vi "test-Coordinate-System-Test1.vi"() -> (3 "All tests passed":bool)   [LabVIEW 2019]
uses:
  <vilib>/Rock Robotics/WPI/ThirdParty/JAS_Junk/TrajLib/CoordAxis_N.vi
  <vilib>/Rock Robotics/WPI/ThirdParty/JAS_Junk/TrajLib/CoordAxis_W.vi
  <vilib>/Rock Robotics/WPI/ThirdParty/JAS_Junk/TrajLib/CoordAxis_U.vi
  <vilib>/Rock Robotics/WPI/ThirdParty/JAS_Junk/TrajLib/CoordSystem_New.vi
  <vilib>/Rock Robotics/WPI/ThirdParty/JAS_Junk/TrajLib/CoordAxis_E.vi
  <vilib>/Rock Robotics/WPI/ThirdParty/JAS_Junk/TrajLib/CoordAxis_D.vi
  <vilib>/Rock Robotics/WPI/ThirdParty/JAS_Junk/TrajLib/Conv_Deg_Radians.vi
  <vilib>/Rock Robotics/WPI/ThirdParty/JAS_Junk/TrajLib/Quaternion_New.vi
  <vilib>/Rock Robotics/WPI/ThirdParty/JAS_Junk/TrajLib/Translation3d_Create.vi
  <vilib>/Rock Robotics/WPI/ThirdParty/JAS_Junk/TrajLib/Pose3d_New_Trans3dRot3d.vi
  <vilib>/Rock Robotics/WPI/ThirdParty/JAS_Junk/TrajLib/Rotation3d_Minus.vi
  <vilib>/Rock Robotics/WPI/ThirdParty/JAS_Junk/TrajLib/Translation3d_Create_Default.vi
  <vilib>/Rock Robotics/WPI/ThirdParty/JAS_Junk/TrajLib/Pose3d_RelativeTo.vi
  <vilib>/Rock Robotics/WPI/ThirdParty/JAS_Junk/TrajLib/Translation3d_Equals.vi
  <vilib>/Rock Robotics/WPI/ThirdParty/JAS_Junk/TrajLib/Rotation3d_Equals.vi
  <vilib>/Rock Robotics/WPI/ThirdParty/JAS_Junk/TrajLib/Pose3d_getTranslation3d.vi
  <vilib>/Rock Robotics/WPI/ThirdParty/JAS_Junk/TrajLib/Pose3d_getRotation3d.vi
  <vilib>/Rock Robotics/WPI/ThirdParty/JAS_Junk/TrajLib/CoordAxis_New.vi
  <vilib>/Rock Robotics/WPI/ThirdParty/JAS_Junk/TrajLib/MatBuilder_Create.vi
  <vilib>/Rock Robotics/WPI/ThirdParty/JAS_Junk/TrajLib/Matrix_AssignBlock.vi
  <vilib>/Rock Robotics/WPI/ThirdParty/JAS_Junk/TrajLib/Matrix_Transpose.vi
  <vilib>/Rock Robotics/WPI/ThirdParty/JAS_Junk/TrajLib/Matrix_Ident.vi
  <vilib>/Rock Robotics/WPI/ThirdParty/JAS_Junk/TrajLib/Matrix_IsEqual.vi
  <vilib>/Analysis/baseanly.llb/A x B.vi
  <vilib>/Analysis/baseanly.llb/Real A x B.vi
  <vilib>/Rock Robotics/WPI/ThirdParty/JAS_Junk/TrajLib/Rotation3d_Create_Quaternion.vi
  <vilib>/Rock Robotics/WPI/ThirdParty/JAS_Junk/TrajLib/Rotation3d_UnaryMinus.vi
  <vilib>/Rock Robotics/WPI/ThirdParty/JAS_Junk/TrajLib/Rotation3d_RotateBy.vi
  <vilib>/Rock Robotics/WPI/ThirdParty/JAS_Junk/TrajLib/Transform3d_Create_Pose3dPose3d.vi
  <vilib>/Rock Robotics/WPI/ThirdParty/JAS_Junk/TrajLib/Transform3d_GetRotation3d.vi
  <vilib>/Rock Robotics/WPI/ThirdParty/JAS_Junk/TrajLib/Transform3d_GetTranslation3d.vi
  <vilib>/Rock Robotics/WPI/ThirdParty/JAS_Junk/TrajLib/Rotation3d_GetQuaterion.vi
  <vilib>/Rock Robotics/WPI/ThirdParty/JAS_Junk/TrajLib/Quaternion_Equals.vi
  <vilib>/Rock Robotics/WPI/ThirdParty/JAS_Junk/TrajLib/MatrixHelper_CoerceSize.vi
  <vilib>/Rock Robotics/WPI/ThirdParty/JAS_Junk/TrajLib/Quaternion_Normalize.vi
  <vilib>/Rock Robotics/WPI/ThirdParty/JAS_Junk/TrajLib/Quaternion_Inverse.vi
  <vilib>/Rock Robotics/WPI/ThirdParty/JAS_Junk/TrajLib/Quaternion_Times.vi
  <vilib>/Rock Robotics/WPI/ThirdParty/JAS_Junk/TrajLib/Transform3d_Create_Trans3dRot3d.vi
  <vilib>/Rock Robotics/WPI/ThirdParty/JAS_Junk/TrajLib/Translation3d_Minus.vi
  <vilib>/Rock Robotics/WPI/ThirdParty/JAS_Junk/TrajLib/Translation3d_RotateBy.vi
  <vilib>/Rock Robotics/WPI/ThirdParty/JAS_Junk/TrajLib/Quaternion_New_Default.vi
  <vilib>/Rock Robotics/WPI/ThirdParty/JAS_Junk/TrajLib/Quaternion_Get_All.vi
  <vilib>/Analysis/7linalg.llb/Create Special Matrix.vi
  <vilib>/Analysis/7linalg.llb/Create Special Real Matrix.vi
  <vilib>/Analysis/Matrix/Numeric/Conversions/Array To Matrix.vi
  <vilib>/Analysis/Matrix/Numeric/Conversions/Array To Matrix - RA.vi
  <vilib>/Rock Robotics/WPI/ThirdParty/JAS_Junk/TrajLib/Trajectory_Library.lvlib
panel:
  out "Test 4":bool
  out "Test 3":bool
  out "Test 2":bool
  out "Test 1":bool
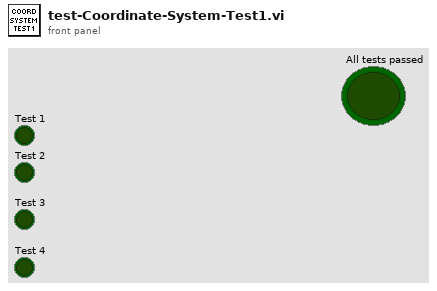
[diagram p1: front panel]
types:
  T1 = typedef "Trajectory_Library.lvlib/ROTATION3D.ctl" = cluster{"Q_quaternion":T2}
  T2 = typedef "Trajectory_Library.lvlib/QUATERNION.ctl" = cluster{"R":dbl, "V":dbl[]}
  T3 = typedef "Trajectory_Library.lvlib/POSE3D.ctl" = cluster{"Translation3d":T4, "Rotation3d":T1}
  T4 = typedef "Trajectory_Library.lvlib/TRANSLATION3D.ctl" = cluster{"X":dbl, "Y":dbl, "Z":dbl}
  T5 = typedef "Trajectory_Library.lvlib/COORDINATE_SYSTEM.ctl" = cluster{"Rotation":T1}
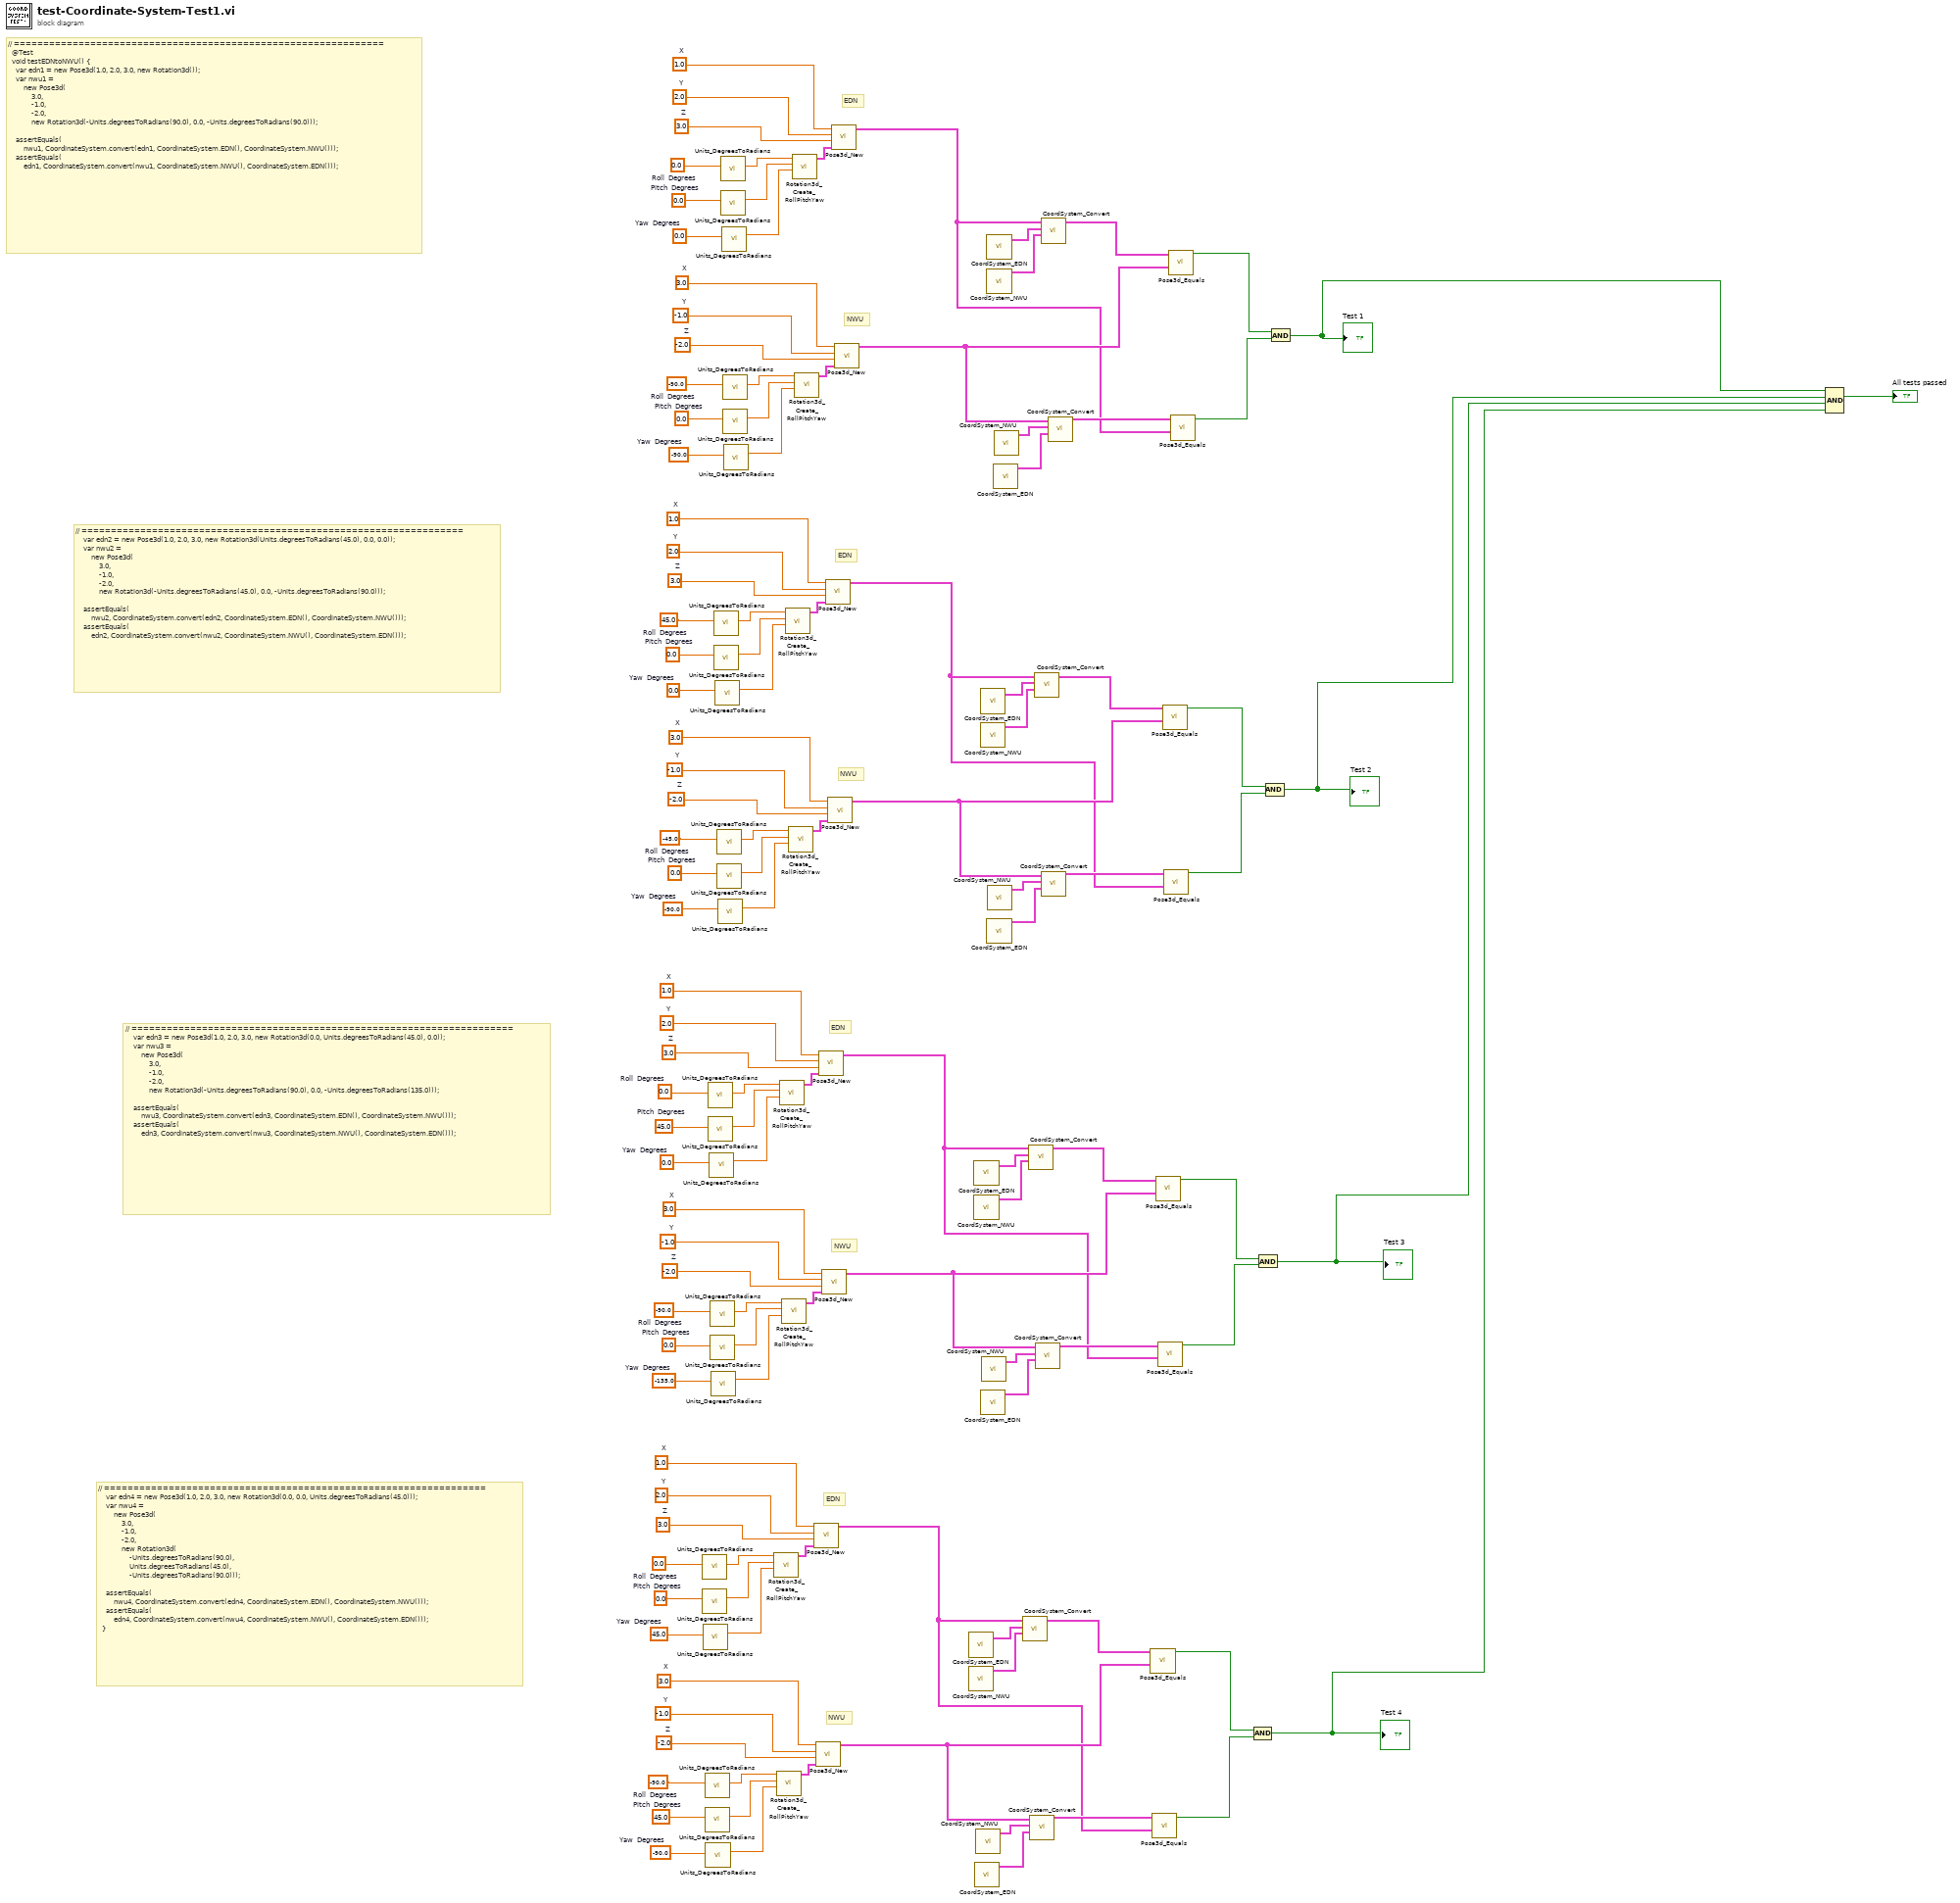
[diagram p0: block diagram]
diagram:
  w22 = 3.0  # X
  w21 = -1.0  # Y
  w20 = -2.0  # Z
  w14 = -90.0  # Roll  Degrees
  w15 = 45.0  # Pitch  Degrees
  w16 = -90.0  # Yaw  Degrees
  w32 = 1.0  # X
  w31 = 2.0  # Y
  w30 = 3.0  # Z
  w24 = 0.0  # Roll  Degrees
  w25 = 0.0  # Pitch  Degrees
  w26 = 45.0  # Yaw  Degrees
  w52 = 3.0  # X
  w51 = -1.0  # Y
  w50 = -2.0  # Z
  w44 = -90.0  # Roll  Degrees
  w45 = 0.0  # Pitch  Degrees
  w46 = -135.0  # Yaw  Degrees
  w62 = 1.0  # X
  w61 = 2.0  # Y
  w60 = 3.0  # Z
  w54 = 0.0  # Roll  Degrees
  w55 = 45.0  # Pitch  Degrees
  w56 = 0.0  # Yaw  Degrees
  w82 = 3.0  # X
  w81 = -1.0  # Y
  w80 = -2.0  # Z
  w74 = -45.0  # Roll  Degrees
  w75 = 0.0  # Pitch  Degrees
  w76 = -90.0  # Yaw  Degrees
  w92 = 1.0  # X
  w91 = 2.0  # Y
  w90 = 3.0  # Z
  w84 = 45.0  # Roll  Degrees
  w85 = 0.0  # Pitch  Degrees
  w86 = 0.0  # Yaw  Degrees
  w114 = 3.0  # X
  w113 = -1.0  # Y
  w112 = -2.0  # Z
  w106 = -90.0  # Roll  Degrees
  w107 = 0.0  # Pitch  Degrees
  w108 = -90.0  # Yaw  Degrees
  w124 = 1.0  # X
  w123 = 2.0  # Y
  w122 = 3.0  # Z
  w116 = 0.0  # Roll  Degrees
  w117 = 0.0  # Pitch  Degrees
  w118 = 0.0  # Yaw  Degrees
  # "// =================================================================\n    var edn2 = new Pose3d(1.0, 2.0, 3.0, new Rotation3d(Units.degreesToRadians(45.0), 0.0, 0.0));\n    var nwu2 =\n        new Pose3d(\n            3.0,\n            -1.0,\n            -2.0,\n            new Rotation3d(-Units.degreesToRadians(45.0), 0.0, -Units.degreesToRadians(90.0)));\n\n    assertEquals(\n        nwu2, CoordinateSystem.convert(edn2, CoordinateSystem.EDN(), CoordinateSystem.NWU()));\n    assertEquals(\n        edn2, CoordinateSystem.convert(nwu2, CoordinateSystem.NWU(), CoordinateSystem.EDN()));"
  # "// =================================================================\n    var edn3 = new Pose3d(1.0, 2.0, 3.0, new Rotation3d(0.0, Units.degreesToRadians(45.0), 0.0));\n    var nwu3 =\n        new Pose3d(\n            3.0,\n            -1.0,\n            -2.0,\n            new Rotation3d(-Units.degreesToRadians(90.0), 0.0, -Units.degreesToRadians(135.0)));\n\n    assertEquals(\n        nwu3, CoordinateSystem.convert(edn3, CoordinateSystem.EDN(), CoordinateSystem.NWU()));\n    assertEquals(\n        edn3, CoordinateSystem.convert(nwu3, CoordinateSystem.NWU(), CoordinateSystem.EDN()));"
  # "// =================================================================\n    var edn4 = new Pose3d(1.0, 2.0, 3.0, new Rotation3d(0.0, 0.0, Units.degreesToRadians(45.0)));\n    var nwu4 =\n        new Pose3d(\n            3.0,\n            -1.0,\n            -2.0,\n            new Rotation3d(\n                -Units.degreesToRadians(90.0),\n                Units.degreesToRadians(45.0),\n                -Units.degreesToRadians(90.0)));\n\n    assertEquals(\n        nwu4, CoordinateSystem.convert(edn4, CoordinateSystem.EDN(), CoordinateSystem.NWU()));\n    assertEquals(\n        edn4, CoordinateSystem.convert(nwu4, CoordinateSystem.NWU(), CoordinateSystem.EDN()));\n  }"
  # "NWU"
  # "EDN"
  # "NWU"
  # "EDN"
  # "NWU"
  # "EDN"
  # "NWU"
  # "EDN"
  # "// ===============================================================\n  @Test\n  void testEDNtoNWU() {\n    var edn1 = new Pose3d(1.0, 2.0, 3.0, new Rotation3d());\n    var nwu1 =\n        new Pose3d(\n            3.0,\n            -1.0,\n            -2.0,\n            new Rotation3d(-Units.degreesToRadians(90.0), 0.0, -Units.degreesToRadians(90.0)));\n\n    assertEquals(\n        nwu1, CoordinateSystem.convert(edn1, CoordinateSystem.EDN(), CoordinateSystem.NWU()));\n    assertEquals(\n        edn1, CoordinateSystem.convert(nwu1, CoordinateSystem.NWU(), CoordinateSystem.EDN()));"
  n1 = call <vilib>:"Units_DegreesToRadians.vi"("Degrees"=w24) -> ("Radians"=w27:dbl)  [unwired: 10 in]
  n2 = call <vilib>:"Units_DegreesToRadians.vi"("Degrees"=w25) -> ("Radians"=w28:dbl)  [unwired: 10 in]
  n3 = call <vilib>:"Units_DegreesToRadians.vi"("Degrees"=w26) -> ("Radians"=w29:dbl)  [unwired: 10 in]
  n4 = call <vilib>:"Units_DegreesToRadians.vi"("Degrees"=w14) -> ("Radians"=w17:dbl)  [unwired: 10 in]
  n5 = call <vilib>:"Units_DegreesToRadians.vi"("Degrees"=w15) -> ("Radians"=w18:dbl)  [unwired: 10 in]
  n6 = call <vilib>:"Units_DegreesToRadians.vi"("Degrees"=w16) -> ("Radians"=w19:dbl)  [unwired: 10 in]
  n7 = call <vilib>:"Units_DegreesToRadians.vi"("Degrees"=w54) -> ("Radians"=w57:dbl)  [unwired: 10 in]
  n8 = call <vilib>:"Units_DegreesToRadians.vi"("Degrees"=w55) -> ("Radians"=w58:dbl)  [unwired: 10 in]
  n9 = call <vilib>:"Units_DegreesToRadians.vi"("Degrees"=w56) -> ("Radians"=w59:dbl)  [unwired: 10 in]
  n10 = call <vilib>:"Units_DegreesToRadians.vi"("Degrees"=w44) -> ("Radians"=w47:dbl)  [unwired: 10 in]
  n11 = call <vilib>:"Units_DegreesToRadians.vi"("Degrees"=w45) -> ("Radians"=w48:dbl)  [unwired: 10 in]
  n12 = call <vilib>:"Units_DegreesToRadians.vi"("Degrees"=w46) -> ("Radians"=w49:dbl)  [unwired: 10 in]
  n13 = call <vilib>:"Units_DegreesToRadians.vi"("Degrees"=w84) -> ("Radians"=w87:dbl)  [unwired: 10 in]
  n14 = call <vilib>:"Units_DegreesToRadians.vi"("Degrees"=w85) -> ("Radians"=w88:dbl)  [unwired: 10 in]
  n15 = call <vilib>:"Units_DegreesToRadians.vi"("Degrees"=w86) -> ("Radians"=w89:dbl)  [unwired: 10 in]
  n16 = call <vilib>:"Units_DegreesToRadians.vi"("Degrees"=w74) -> ("Radians"=w77:dbl)  [unwired: 10 in]
  n17 = call <vilib>:"Units_DegreesToRadians.vi"("Degrees"=w75) -> ("Radians"=w78:dbl)  [unwired: 10 in]
  n18 = call <vilib>:"Units_DegreesToRadians.vi"("Degrees"=w76) -> ("Radians"=w79:dbl)  [unwired: 10 in]
  n19 = call <vilib>:"Units_DegreesToRadians.vi"("Degrees"=w116) -> ("Radians"=w119:dbl)  [unwired: 10 in]
  n20 = call <vilib>:"Units_DegreesToRadians.vi"("Degrees"=w117) -> ("Radians"=w120:dbl)  [unwired: 10 in]
  n21 = call <vilib>:"Units_DegreesToRadians.vi"("Degrees"=w118) -> ("Radians"=w121:dbl)  [unwired: 10 in]
  n22 = call <vilib>:"Units_DegreesToRadians.vi"("Degrees"=w106) -> ("Radians"=w109:dbl)  [unwired: 10 in]
  n23 = call <vilib>:"Units_DegreesToRadians.vi"("Degrees"=w107) -> ("Radians"=w110:dbl)  [unwired: 10 in]
  n24 = call <vilib>:"Units_DegreesToRadians.vi"("Degrees"=w108) -> ("Radians"=w111:dbl)  [unwired: 10 in]
  n25 = call <vilib>:"Rotation3d_Create_RollPitchYaw.vi"("Yaw"=w29, "Pitch"=w28, "Roll"=w27) -> ("Rotation3d"=w33:T1)  [unwired: 8 in]
  n26 = call <vilib>:"Rotation3d_Create_RollPitchYaw.vi"("Yaw"=w19, "Pitch"=w18, "Roll"=w17) -> ("Rotation3d"=w23:T1)  [unwired: 8 in]
  n27 = call <vilib>:"Rotation3d_Create_RollPitchYaw.vi"("Yaw"=w59, "Pitch"=w58, "Roll"=w57) -> ("Rotation3d"=w63:T1)  [unwired: 8 in]
  n28 = call <vilib>:"Rotation3d_Create_RollPitchYaw.vi"("Yaw"=w49, "Pitch"=w48, "Roll"=w47) -> ("Rotation3d"=w53:T1)  [unwired: 8 in]
  n29 = call <vilib>:"Rotation3d_Create_RollPitchYaw.vi"("Yaw"=w89, "Pitch"=w88, "Roll"=w87) -> ("Rotation3d"=w93:T1)  [unwired: 8 in]
  n30 = call <vilib>:"Rotation3d_Create_RollPitchYaw.vi"("Yaw"=w79, "Pitch"=w78, "Roll"=w77) -> ("Rotation3d"=w83:T1)  [unwired: 8 in]
  n31 = call <vilib>:"Rotation3d_Create_RollPitchYaw.vi"("Yaw"=w121, "Pitch"=w120, "Roll"=w119) -> ("Rotation3d"=w125:T1)  [unwired: 8 in]
  n32 = call <vilib>:"Rotation3d_Create_RollPitchYaw.vi"("Yaw"=w111, "Pitch"=w110, "Roll"=w109) -> ("Rotation3d"=w115:T1)  [unwired: 8 in]
  n33 = call <vilib>:"Pose3d_New.vi"("Rotation3d"=w33, "z"=w30, "Y"=w31, "X"=w32) -> ("out Pose3d"=w6:T3)  [unwired: 7 in]
  n34 = call <vilib>:"Pose3d_New.vi"("Rotation3d"=w23, "z"=w20, "Y"=w21, "X"=w22) -> ("out Pose3d"=w8:T3)  [unwired: 7 in]
  n35 = call <vilib>:"Pose3d_New.vi"("Rotation3d"=w63, "z"=w60, "Y"=w61, "X"=w62) -> ("out Pose3d"=w36:T3)  [unwired: 7 in]
  n36 = call <vilib>:"Pose3d_New.vi"("Rotation3d"=w53, "z"=w50, "Y"=w51, "X"=w52) -> ("out Pose3d"=w38:T3)  [unwired: 7 in]
  n37 = call <vilib>:"Pose3d_New.vi"("Rotation3d"=w93, "z"=w90, "Y"=w91, "X"=w92) -> ("out Pose3d"=w66:T3)  [unwired: 7 in]
  n38 = call <vilib>:"Pose3d_New.vi"("Rotation3d"=w83, "z"=w80, "Y"=w81, "X"=w82) -> ("out Pose3d"=w68:T3)  [unwired: 7 in]
  n39 = call <vilib>:"Pose3d_New.vi"("Rotation3d"=w125, "z"=w122, "Y"=w123, "X"=w124) -> ("out Pose3d"=w98:T3)  [unwired: 7 in]
  n40 = call <vilib>:"Pose3d_New.vi"("Rotation3d"=w115, "z"=w112, "Y"=w113, "X"=w114) -> ("out Pose3d"=w100:T3)  [unwired: 7 in]
  n41 = call <vilib>:"CoordSystem_EDN.vi"() -> ("out Coordinate System"=w13:T5)  [unwired: 10 in, 1 out]
  n42 = call <vilib>:"CoordSystem_NWU.vi"() -> ("out Coordinate System"=w12:T5)  [unwired: 10 in, 1 out]
  n43 = call <vilib>:"CoordSystem_EDN.vi"() -> ("out Coordinate System"=w43:T5)  [unwired: 10 in, 1 out]
  n44 = call <vilib>:"CoordSystem_NWU.vi"() -> ("out Coordinate System"=w42:T5)  [unwired: 10 in, 1 out]
  n45 = call <vilib>:"CoordSystem_EDN.vi"() -> ("out Coordinate System"=w10:T5)  [unwired: 10 in, 1 out]
  n46 = call <vilib>:"CoordSystem_NWU.vi"() -> ("out Coordinate System"=w11:T5)  [unwired: 10 in, 1 out]
  n47 = call <vilib>:"CoordSystem_EDN.vi"() -> ("out Coordinate System"=w73:T5)  [unwired: 10 in, 1 out]
  n48 = call <vilib>:"CoordSystem_NWU.vi"() -> ("out Coordinate System"=w72:T5)  [unwired: 10 in, 1 out]
  n49 = call <vilib>:"CoordSystem_EDN.vi"() -> ("out Coordinate System"=w40:T5)  [unwired: 10 in, 1 out]
  n50 = call <vilib>:"CoordSystem_NWU.vi"() -> ("out Coordinate System"=w41:T5)  [unwired: 10 in, 1 out]
  n51 = call <vilib>:"CoordSystem_EDN.vi"() -> ("out Coordinate System"=w105:T5)  [unwired: 10 in, 1 out]
  n52 = call <vilib>:"CoordSystem_NWU.vi"() -> ("out Coordinate System"=w104:T5)  [unwired: 10 in, 1 out]
  n53 = call <vilib>:"CoordSystem_EDN.vi"() -> ("out Coordinate System"=w70:T5)  [unwired: 10 in, 1 out]
  n54 = call <vilib>:"CoordSystem_NWU.vi"() -> ("out Coordinate System"=w71:T5)  [unwired: 10 in, 1 out]
  n55 = call <vilib>:"CoordSystem_EDN.vi"() -> ("out Coordinate System"=w102:T5)  [unwired: 10 in, 1 out]
  n56 = call <vilib>:"CoordSystem_NWU.vi"() -> ("out Coordinate System"=w103:T5)  [unwired: 10 in, 1 out]
  n57 = call <vilib>:"CoordSystem_Convert.vi"("CoordSys To"=w12, "CoordSys From"=w13, "in Pose3d"=w6) -> ("out Converted Pose3d"=w9:T3)  [unwired: 8 in]
  n58 = call <vilib>:"CoordSystem_Convert.vi"("CoordSys To"=w42, "CoordSys From"=w43, "in Pose3d"=w36) -> ("out Converted Pose3d"=w39:T3)  [unwired: 8 in]
  n59 = call <vilib>:"CoordSystem_Convert.vi"("CoordSys To"=w10, "CoordSys From"=w11, "in Pose3d"=w8) -> ("out Converted Pose3d"=w7:T3)  [unwired: 8 in]
  n60 = call <vilib>:"CoordSystem_Convert.vi"("CoordSys To"=w72, "CoordSys From"=w73, "in Pose3d"=w66) -> ("out Converted Pose3d"=w69:T3)  [unwired: 8 in]
  n61 = call <vilib>:"CoordSystem_Convert.vi"("CoordSys To"=w40, "CoordSys From"=w41, "in Pose3d"=w38) -> ("out Converted Pose3d"=w37:T3)  [unwired: 8 in]
  n62 = call <vilib>:"CoordSystem_Convert.vi"("CoordSys To"=w104, "CoordSys From"=w105, "in Pose3d"=w98) -> ("out Converted Pose3d"=w101:T3)  [unwired: 8 in]
  n63 = call <vilib>:"CoordSystem_Convert.vi"("CoordSys To"=w70, "CoordSys From"=w71, "in Pose3d"=w68) -> ("out Converted Pose3d"=w67:T3)  [unwired: 8 in]
  n64 = call <vilib>:"CoordSystem_Convert.vi"("CoordSys To"=w102, "CoordSys From"=w103, "in Pose3d"=w100) -> ("out Converted Pose3d"=w99:T3)  [unwired: 8 in]
  n65 = call <vilib>:"Pose3d_Equals.vi"("other Pose3d"=w8, "in Pose3d"=w9) -> ("Equals"=w5:bool)  [unwired: 9 in]
  n66 = call <vilib>:"Pose3d_Equals.vi"("other Pose3d"=w6, "in Pose3d"=w7) -> ("Equals"=w4:bool)  [unwired: 9 in]
  n67 = call <vilib>:"Pose3d_Equals.vi"("other Pose3d"=w38, "in Pose3d"=w39) -> ("Equals"=w35:bool)  [unwired: 9 in]
  n68 = call <vilib>:"Pose3d_Equals.vi"("other Pose3d"=w36, "in Pose3d"=w37) -> ("Equals"=w34:bool)  [unwired: 9 in]
  n69 = call <vilib>:"Pose3d_Equals.vi"("other Pose3d"=w68, "in Pose3d"=w69) -> ("Equals"=w65:bool)  [unwired: 9 in]
  n70 = call <vilib>:"Pose3d_Equals.vi"("other Pose3d"=w66, "in Pose3d"=w67) -> ("Equals"=w64:bool)  [unwired: 9 in]
  n71 = call <vilib>:"Pose3d_Equals.vi"("other Pose3d"=w100, "in Pose3d"=w101) -> ("Equals"=w97:bool)  [unwired: 9 in]
  n72 = call <vilib>:"Pose3d_Equals.vi"("other Pose3d"=w98, "in Pose3d"=w99) -> ("Equals"=w96:bool)  [unwired: 9 in]
  n73 = Compound Arithmetic op=AND(w5, w4) -> (w1:bool)
  "Test 4" <- w1
  n74 = Compound Arithmetic op=AND(w35, w34) -> (w2:bool)
  "Test 3" <- w2
  n75 = Compound Arithmetic op=AND(w65, w64) -> (w3:bool)
  "Test 2" <- w3
  n76 = Compound Arithmetic op=AND(w97, w96) -> (w94:bool)
  "Test 1" <- w94
  n77 = Compound Arithmetic op=AND(w94, w3, w2, w1) -> (→"All tests passed":bool)
